vi "StepRealtime_IP9.vi"() -> ()   [LabVIEW 2014]
doc: "This VI was generated automatically using the FPGA Wizard. You can modify the VI normally."
uses:
  <vilib>/Platform/TimedLoop/XDataNode/timing_clust.ctl
  <vilib>/Platform/TimedLoop/XDataNode/nitl_modes.ctl
  <vilib>/Platform/TimedLoop/XDataNode/wakeup.ctl
  <vilib>/FPGAPlugInAG/sbRIO-9632/niLvFpga_Open_sbRIO-9632.vi
  <vilib>/rvi/interface/common/dynamic/niFpgaDynamicAddResources.vi
  <vilib>/FPGAPlugInAG/Dynamic/niLvFpga_Reset_Dynamic.vi
  <vilib>/FPGAPlugInAG/Dynamic/niLvFpga_Run_Dynamic.vi
  <vilib>/Utility/error.llb/Error Cluster From Error Code.vi
  <vilib>/rvi/errors/niLvFpgaAdjustHostInterfaceError.vi
  <vilib>/FPGAPlugInAG/Dynamic/niLvFpga_Close_Dynamic.vi
  <vilib>/rvi/interface/nirviOpenFPGA/nirviOpenFPGA.xnode
  FPGA Bitfiles/PPDControlLab3_FPGATarget_IP9.lvbitx
  SYSID_FPGA2.vi
  <vilib>/rvi/interface/nirviMethod/nirviMethod.xnode
  <vilib>/Platform/TimedLoop/XDataNode/XDataNode.xnode
  <vilib>/rvi/interface/nirviReadWriteControl/nirviReadWriteControl.xnode
  <vilib>/rvi/interface/nirviCloseFPGA/nirviCloseFPGA.xnode
  SysIDRealtime.lvlib
  <vilib>/rvi/interface/Simulation/niFpgaSimulationCallBeginRW.vi
  <vilib>/Platform/TimedLoop/XDataNode/XDNodeRunTimeDep.lvlib
  NiFpgaLv.dll
panel:
  out "fixed-point":fxp<+/-,20,5>
  out "Ratio":fxp<+/-,32,7>
  in  "Gain":fxp<+/-,32,7>=0.006999999284744263
  in  "Radio Buttons":enum32{"Radio Selection 1", "Radio Selection 2"}(radio)
  in  "OK Button":bool
  out "Step Response":dynamicdata(graph)=[{"t0"=timestamp(0 s since 1904-01-01), "dt"=1.0, "Y"=array[2048 elements]}, {"t0"=timestamp(0 s since 1904-01-01), "dt"=1.0, "Y"=array[2048 elements]}, {"t0"=timestamp(0 s since 1904-01-01), "dt"=1.0, "Y"=array[2048 elements]}]
  in  "samples":i32=2048
  in  "Reference":i32=100000
  in  "Quad Reset":bool=TRUE
  in  "DGain":fxp<+/-,32,7>
  in  "PGain":fxp<+/-,32,7>
  out "Amp In":dbl[](graph)
  out "Amp Cpmmand":fxp<+/-,20,5>
  out "Iteration Duration":i64
  out "Position":i32[](graph)
  in  "Control Rate (ticks)":u32=10000
  in  "Period (us)":i64=1000
  out "Finished Late? [i-1]":bool
  out "quad saved (Port0/DIO0,Port0/DIO1)":cluster{"Position":i32, "Index Count":u16}
  out "quad pos (Port0/DIO0,Port0/DIO1)":i32
  out "Late? Latched":bool
  in  "Local Stop 0":bool
  in  "Start 0":bool
  in  "Loop Rate (Hz)":dbl=100000.0
  out "Calculated Rate (Hz)":dbl
  out "error out":errorcluster
  in  "Global Stop":bool
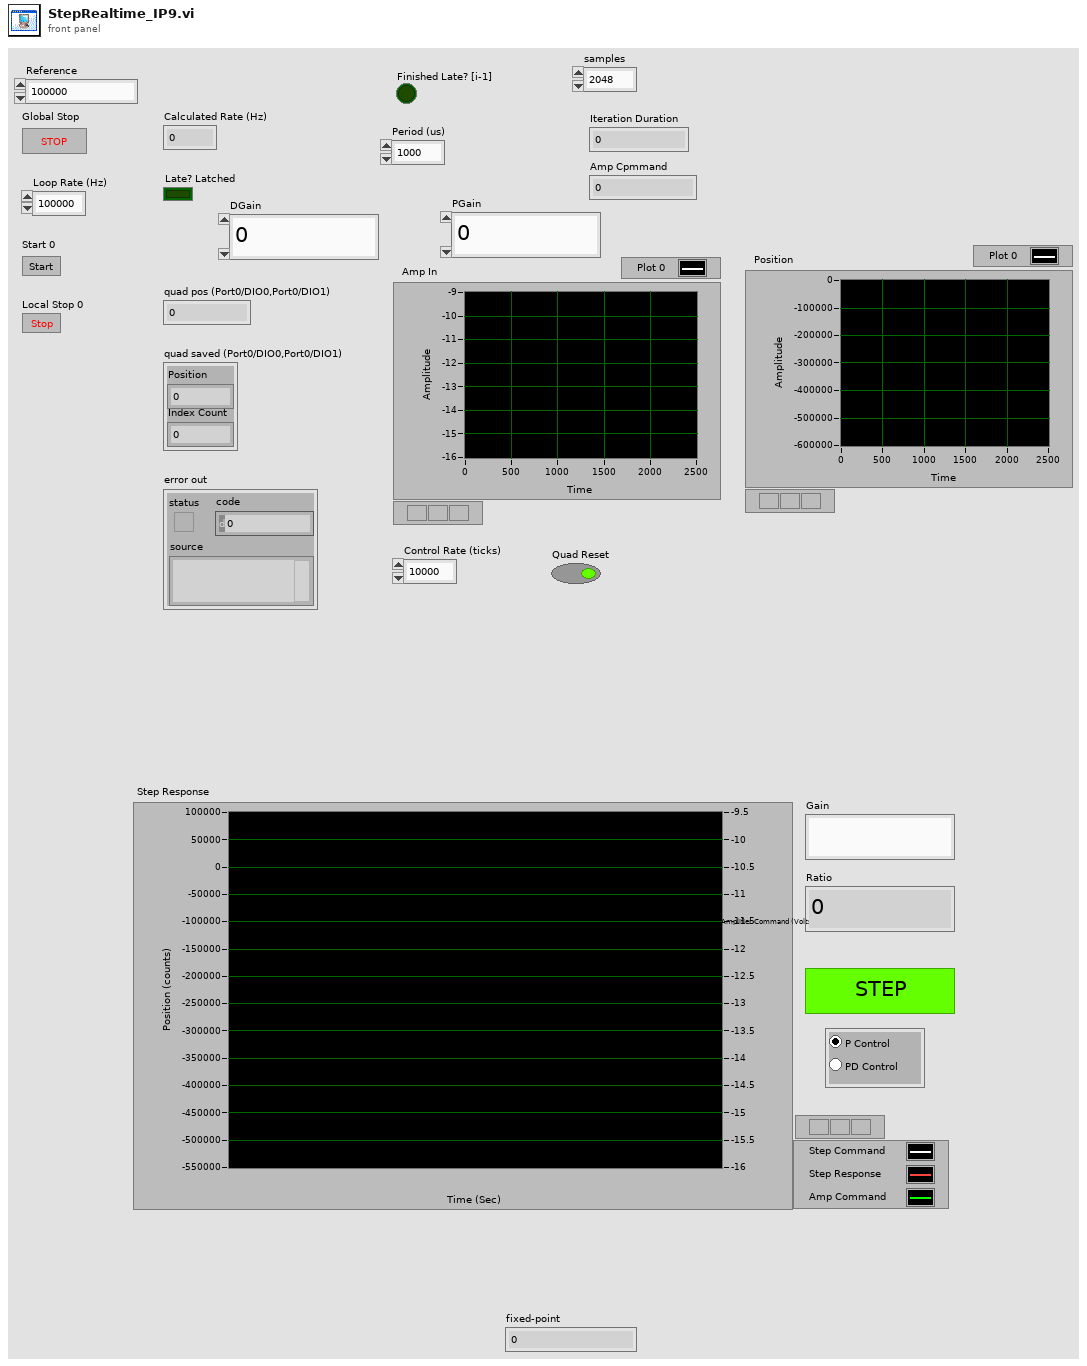
[diagram p1: front panel]
types:
  T1 = typedef "XDNodeRunTimeDep.lvlib/timing_clust.ctl" = cluster{"Expected End [f-1]":u64, "Actual End [f-1]":u64, "Finished Late? [f-1]":bool, "Expected End [i-1]":u64, "Actual End [i-1]":u64, "Finished Late? [i-1]":bool, "Expected Start [i]":u64, "Actual Start [i]":u64, "Expected Start [f]":u64, "Actual Start [f]":u64, "Source Name":string, "Structure Name":string, "Period":i64, "Deadline":i64, "Offset":i64, "Start":i64, "Priority":i32, "Timeout":i32, "Mode":T2, "Wakeup Reason":T3, "Error":errorcluster, "Source Type":string, "Secondary Source Type":string, "Global End Time":u64, "Global Start Time":u64, "Frame Duration":u64, "Iteration Duration":u64, "Assigned CPU":i32, "I/O Scan Engine Mode":u32}
  T2 = typedef "XDNodeRunTimeDep.lvlib/nitl_modes.ctl" = enum32{"No Change", "Process missed periods, maintain original phase", "Discard missed periods, maintain original phase", "Process missed periods, ignore original phase", "Discard missed periods, ignore original phase"}
  T3 = typedef "XDNodeRunTimeDep.lvlib/wakeup.ctl" = enum32{"Normal", "Aborted", "Asynchronous wakeup", "Timing source error", "Timed loop error", "Timeout"}
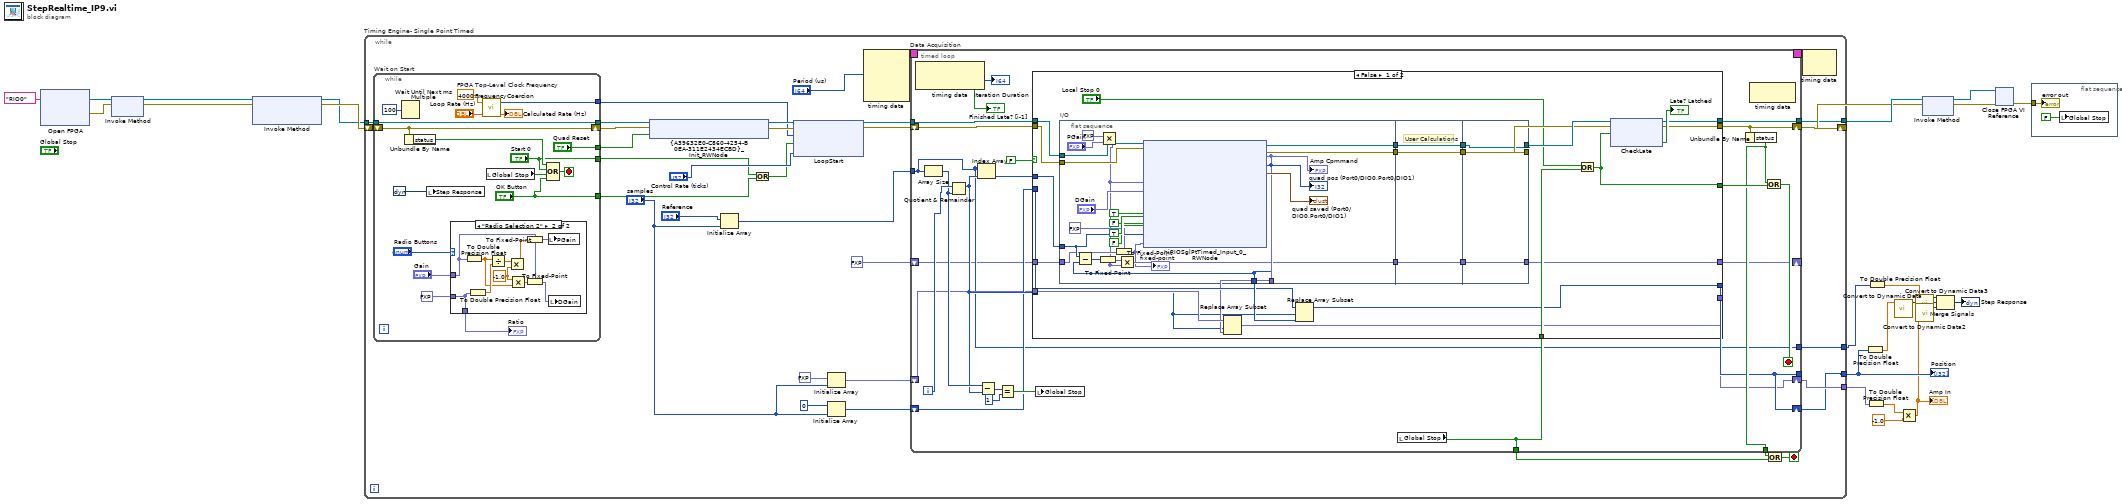
[diagram p0: block diagram]
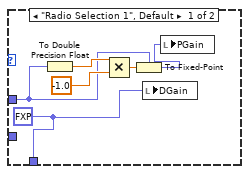
[diagram p3: hidden frame]
diagram:
  n1 = xnode ("Open FPGA")("resource name"=tag "RIO0") -> ("FPGA VI Reference Out"=w22:refnum<k20>, "error out"=w23:errorcluster)  [unwired: 1 in]
  n2 = xnode ("Invoke Method")("FPGA VI Reference In"=w22, "error in"=w23) -> ("FPGA VI Reference Out"=w5:refnum<k20>, "error out"=w4:errorcluster)
  n3 = xnode ("Invoke Method")("FPGA VI Reference In"=w5, "error in"=w4) -> ("FPGA VI Reference Out"=w10:refnum<k20>, "error out"=w24:errorcluster)  [unwired: 1 in]
  n4 = while "Timing Engine- Single Point Timed" {
    tunnel: w10 -> [w54]
    shift-right: [w53] -> w8
    shift-left: w24 -> [w57]
    tunnel: [w35] -> w16
    tunnel: [w36] -> w20
    tunnel: [w30] -> w14
    tunnel: [w26] -> w9
    stop <- w48 stop-if-true
    n5 = while "Wait on Start" {
      tunnel: w54 -> [w165]
      tunnel: [w165] -> w52
      tunnel: [w157] -> w45
      tunnel: ["Start 0"] -> w29
      shift-right: [w159] -> w51
      shift-left: w57 -> [w159]
      tunnel: ["Quad Reset"] -> w34
      tunnel: ["OK Button"] -> w28
      stop <- w166 stop-if-true
      w160 = 40000000.0  # FPGA Top-Level Clock Frequency
      n6 = Wait Until Next ms Multiple(millisecond multiple=u32 100) -> ()  [unwired: 1 out]
      n7 = Unbundle By Name(w159) -> ("status"=w158:bool)
      n8 = local write "Step Response"(dynamicdata [] ("Step Response")) -> ()
      n9 = case shown="\"Radio Selection 2\"" "Radio Buttons" {
        tunnel: "Gain" -> [w168 w174]
        tunnel: fxp<+/-,32,7> 40.0 ("Ratio") -> [_ w179]
        tunnel: [w172 w179] -> w150
        frame "Radio Selection 1", Default {
          w172 = fxp<+/-,32,7> 0.0 ("DGain")
          n10 = To Double Precision Float(number=w168) -> (double precision float=w171:dbl)
          n11 = Multiply(x=w171, y=-1.0) -> (x*y=w169:dbl)
          n12 = To Fixed-Point(fixed-point type=w168, number=w169) -> (fixed-point=w167:fxp<+/-,32,7>)
          n13 = local write "DGain"(w172) -> ()
          n14 = local write "PGain"(w167) -> ()
        }
        frame "Radio Selection 2" {
          w177 = -1.0 ("y")
          n15 = To Double Precision Float(number=w174) -> (double precision float=w176:dbl)
          n16 = To Double Precision Float(number=w179) -> (double precision float=w182:dbl)
          n17 = Divide(x=w176, y=w182) -> (x/y=w181:dbl)
          n18 = Multiply(x=w181, y=w177) -> (x*y=w178:dbl)
          n19 = Multiply(x=w177, y=w176) -> (x*y=w175:dbl)
          n20 = To Fixed-Point(fixed-point type=w174, number=w178) -> (fixed-point=w180:fxp<+/-,32,7>)
          n21 = To Fixed-Point(fixed-point type=w174, number=w175) -> (fixed-point=w173:fxp<+/-,32,7>)
          n22 = local write "PGain"(w180) -> ()
          n23 = local write "DGain"(w173) -> ()
        }
      }
      "Ratio" <- w150
      n24 = call "FrequencyCoercion.vi"("Loop Rate (Hz)"="Loop Rate (Hz)", "FPGA Top-Level Clock Frequency"=w160) -> ("Actual Rate (Hz)"=→"Calculated Rate (Hz)":dbl, "FPGA Ticks"=w157:u32)  [unwired: 2 in]
      n25 = local read "Global Stop"() -> (w163:bool)
      n26 = Compound Arithmetic op=OR(w158, "Start 0", w163, "OK Button") -> (w166:bool)
    }
    n27 = xnode ("{A39632E0-C860-4254-B0EA-311E2434ECBD}_Init_RWNode")("FPGA VI Reference In"=w52, "error in"=w51, "quad reset (Port0/DIO0,Port0/DIO1)"=w34) -> ("FPGA VI Reference Out"=w46:refnum<k20>, "error out"=w50:errorcluster)
    n28 = Initialize Array("Reference", "samples") -> (w31:i32[])
    n29 = Or(x=w29, y=w28) -> (x .or. y?=w27:bool)
    n30 = xnode ("LoopStart")("FPGA VI Reference In"=w46, "error in"=w50, "Loop Rate (Ticks)"=w45, "Start 0"=w27, "Control Rate (ticks)"="Control Rate (ticks)") -> ("FPGA VI Reference Out"=w56:refnum<k20>, "error out"=w55:errorcluster)
    n31 = Initialize Array(0 ("quad pos (Port0/DIO0,Port0/DIO1)"), "samples") -> (w39:i32[])
    n32 = Initialize Array(fxp<+/-,20,5> 0.0 ("Amp Cpmmand"), "samples") -> (w37:fxp<+/-,20,5>[])
    n33 = node-c288("Period (us)") -> (w44:T1)  [unwired: 3 in]
    n34 = timed-loop "Data Acquisition" {
      tunnel: w56 -> [w77]
      tunnel: [w79] -> w49
      tunnel: [w78] -> w47
      shift-right: [w82] -> w53
      shift-left: w55 -> [w76]
      timing: w44 -> [_]
      timing-out: [_] -> w43
      tunnel: w31 -> [w61]
      tunnel: [w63] -> _
      shift-right: [w62] -> w36
      shift-left: w37 -> [w64]
      shift-right: [w63] -> w35
      shift-left: w39 -> [w66]
      tunnel: [w61] -> w30
      tunnel: [w60] -> w26
      shift-right: [w59] -> _
      shift-left: fxp<+/-,64,14> 0.0 -> [w58]
      i -> [w73]
      stop <- w80 stop-if-true
      n35 = node-c288() -> (→"Finished Late? [i-1]":bool, →"Iteration Duration":i64)  [unwired: 1 in]
      n36 = Array Size(array=w61) -> (size(s)=w71:i32)
      n37 = Quotient & Remainder(x=w73, y=w71) -> (x-y*floor(x/y)=w67:i32)  [unwired: 1 out]
      n38 = Index Array(array=w61, index=w67) -> (element=w72:i32)
      n39 = Subtract(x=w71, y=w67) -> (x-y=w70:i32)
      n40 = Equal?(x=w70, y=1) -> (x = y?=w68:bool)
      n41 = local write "Global Stop"(w68) -> ()
      n42 = local read "Global Stop"() -> (w79:bool)
      n43 = case "Timeout" shown="False" FALSE {
        tunnel: w77 -> [w107 w142]
        tunnel: w76 -> [w106 w144]
        tunnel: [w100 w144] -> w82
        tunnel: [w102 w143] -> w81
        tunnel: w79 -> [w103 w143]
        tunnel: w72 -> [w92 _]
        tunnel: w67 -> [w94 _]
        tunnel: w66 -> [w98 _]
        tunnel: [w97 _] -> w63
        tunnel: w64 -> [w96 _]
        tunnel: [w93 _] -> w62
        tunnel: [w91 w142] -> w60
        tunnel: [w89 w141] -> w59
        tunnel: w58 -> [w87 w141]
        frame False {
          n44 = flat-sequence "I/O" {
            tunnel: w107 -> [w132]
            tunnel: w106 -> [w134]
            tunnel: [w133] -> w112
            tunnel: [w131] -> w109
            tunnel: [w122] -> w99
            tunnel: [w129] -> w95
            tunnel: w92 -> [w123]
            tunnel: [w118] -> w90
            tunnel: w87 -> [w115]
            tunnel: [w137] -> w111
            tunnel: w112 -> [w136]
            tunnel: w109 -> [w137]
            tunnel: [w136] -> w110
            tunnel: w90 -> [w135]
            tunnel: [w135] -> w88
            tunnel: [w139] -> w105
            tunnel: [w140] -> w108
            tunnel: w111 -> [w140]
            tunnel: w110 -> [w139]
            tunnel: [w138] -> w89
            tunnel: w88 -> [w138]
            frame #0 {
              n45 = Multiply(x=fxp<+/-,32,7> 1.0, y="PGain") -> (x*y=w114:fxp<+/-,64,14>)
              n46 = To Fixed-Point(fixed-point type=fxp<+/-,20,5> 0.0 ("State_Control"), number=w115) -> (fixed-point=w117:fxp<+/-,20,5>)
              "fixed-point" <- w117
              n47 = xnode ("niRIOSglPtTimed_Input_0_RWNode")("FPGA VI Reference In"=w132, "error in"=w134, "PGain"=w114, "DGain"="DGain", "Amp Enable"=TRUE, "Amp Reset"=FALSE, "Brake"=TRUE, "quad reset (Port0/DIO0,Port0/DIO1)"=FALSE, "Reference"=w123, "State_Control"=w117) -> ("FPGA VI Reference Out"=w131:refnum<k20>, "error out"=w133:errorcluster, "Amp Cpmmand"=w129:fxp<+/-,20,5>, "Stage Position"=w122:i32, "quad saved (Port0/DIO0,Port0/DIO1)"=→"quad saved (Port0/DIO0,Port0/DIO1)":cluster{"Position":i32, "Index Count":u16})
              "quad pos (Port0/DIO0,Port0/DIO1)" <- w122
              "Amp Cpmmand" <- w129
              n48 = Subtract(x=w123, y=w122) -> (x-y=w120:i32)
              n49 = To Fixed-Point(fixed-point type=w114, number=w120) -> (fixed-point=w121:fxp<+/-,64,14>)
              n50 = Multiply(x=w121, y=w114) -> (x*y=w118:fxp<+/-,64,26>)
            }
            frame #1 {
              # "User Calculations"
            }
            frame #2 {
            }
          }
          n51 = Replace Array Subset(array=w96, new element=w95, index=w94) -> (w93:fxp<+/-,20,5>[])
          n52 = Replace Array Subset(array=w98, new element=w99, index=w94) -> (w97:i32[])
          n53 = Or(x="Local Stop 0", y=w103) -> (x .or. y?=w102:bool)
          n54 = xnode ("CheckLate")("FPGA VI Reference In"=w108, "error in"=w105, "Local Stop 0"=w102) -> ("FPGA VI Reference Out"=w91:refnum<k20>, "error out"=w100:errorcluster, "Late? Latched"=→"Late? Latched":bool)
        }
        frame True {
          # "Timeout waiting for an interrupt. This case checks the state of the global stop.\nIf global stop is not set, then loop around to wait for an interrupt again."
        }
      }
      n55 = Unbundle By Name(w82) -> ("status"=w78:bool)
      n56 = node-c288() -> ()  [unwired: 1 in, 1 out]
      n57 = Or(x=w78, y=w81) -> (x .or. y?=w80:bool)
    }
    n58 = Or(x=w47, y=w49) -> (x .or. y?=w48:bool)
    n59 = node-c288(w43) -> ()  [unwired: 1 out]
  }
  "Position" <- w16
  n60 = To Double Precision Float(number=w16) -> (double precision float=w15:dbl[])
  n61 = To Double Precision Float(number=w20) -> (double precision float=w2:dbl[])
  n62 = To Double Precision Float(number=w14) -> (double precision float=w13:dbl[])
  n63 = call "Convert to Dynamic Data"("Array"=w15) -> ("Dynamic Data Type"=w18:dynamicdata)  [unwired: 3 in]
  n64 = Multiply(x=w2, y=-1.0) -> (x*y=w1:dbl[])
  "Amp In" <- w1
  n65 = call "Convert to Dynamic Data3"("Array"=w13) -> ("Dynamic Data Type"=w12:dynamicdata)  [unwired: 3 in]
  n66 = call "Convert to Dynamic Data2"("Array"=w1) -> ("Dynamic Data Type"=w17:dynamicdata)  [unwired: 3 in]
  n67 = xnode "Invoke Method"("FPGA VI Reference In"=w9, "error in"=w8) -> ("FPGA VI Reference Out"=w7:refnum<k20>, "error out"=w6:errorcluster)
  n68 = Merge Signals(w12, w18, w17) -> (→"Step Response":dynamicdata)
  n69 = xnode ("Close FPGA VI Reference")("FPGA VI Reference In"=w7, "error in"=w6) -> ("error out"=w21:errorcluster)
  n70 = flat-sequence {
    tunnel: w21 -> [w184]
    frame #0 {
      n71 = local write "Global Stop"(FALSE ("Global Stop")) -> ()
      "error out" <- w184
    }
  }
